vi "ExcelInertColumns.vi"(8 "error in (no error)":errorcluster, 9 "start (0, 0)":cluster{"row":i32, "column":i32}, 10 "Numeric":i32, 11 "report in":refnum<class "NI_report.lvclass">) -> (0 "error out":errorcluster, 3 "report out":refnum<class "NI_report.lvclass">)   [LabVIEW 2012]
uses:
  <vilib>/Utility/NIReport.llb/NI_report.lvclass
  <vilib>/Utility/NIReport.llb/Excel/NI_Excel.lvclass
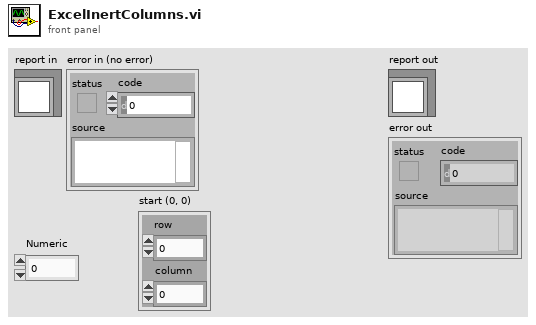
[diagram p1: front panel]
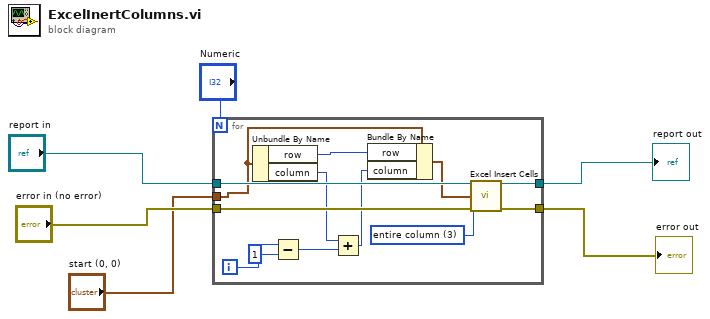
[diagram p0: block diagram]
diagram:
  n1 = for {
    N: "Numeric" -> [_]
    tunnel: "report in" -> [w19]
    tunnel: "error in (no error)" -> [w18]
    tunnel: [w17] -> w4
    tunnel: [w16] -> w3
    tunnel: "start (0, 0)" -> [w12]
    i -> [w15]
    w10 = u16 3 items=["shift cells right", "shift cells down", "entire row", "entire column"] ("mode (entire row)")
    n2 = Unbundle By Name(w12) -> ("row"=w9:i32, "column"=w8:i32)
    n3 = Subtract(x=w15, y=1) -> (x-y=w13:i32)
    n4 = Add(x=w8, y=w13) -> (x+y=w7:i32)
    n5 = Bundle By Name(cluster=w12, "row"=w9, "column"=w7) -> (w11:cluster{"row":i32, "column":i32})
    n6 = call <vilib>:"Excel Insert Cells.vi"("report in"=w19, "mode (entire row)"=w10, "start (0, 0)"=w11, "error in (no error)"=w18) -> ("report out"=w17:refnum<class "NI_report.lvclass">, "error out"=w16:errorcluster)  [unwired: 10 in]
  }
  "report out" <- w4
  "error out" <- w3
